vi "Merge Error.vi"(10 "Error":errorcluster) -> (3 "Merge Error Msg out":refnum<class "Merge Error Msg.lvclass">)   [LabVIEW 2021, in "Merge Error.lvlib" / "Merge Error Msg.lvclass"]
uses:
  Merge Error Msg.lvclass
  Merge Error Msg.lvclass/Merge Error Msg.ctl
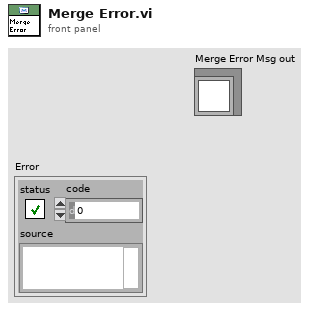
[diagram p1: front panel]
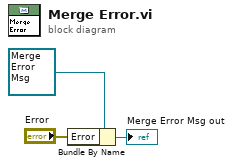
[diagram p0: block diagram]
diagram:
  n1 = Bundle By Name(cluster=refnum<class "Merge Error Msg.lvclass"> refnum ("Error Msg Strategy out"), "Error"="Error") -> (→"Merge Error Msg out":refnum<class "Merge Error Msg.lvclass">)
